vi "Calculate Frequency Response.vi"(9 "Amplitudes":dbl[](array[numeric]), 11 "Frequencies":dbl[](array[numeric])) -> (3 "Frequency response @ 1KHz":dbl[](array[numeric]))   [LabVIEW 2021, in "audio_frequencyResponseMeasurement.lvlib"]
uses:
  audio_frequencyResponseMeasurement.lvlib
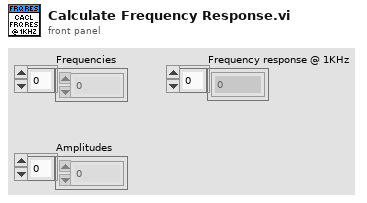
[diagram p1: front panel]
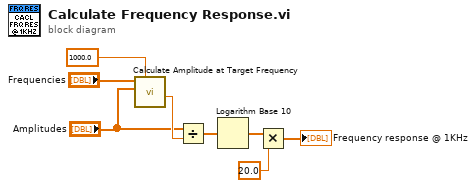
[diagram p0: block diagram]
diagram:
  n1 = call "Calculate Amplitude at Target Frequency.vi"("Target frequency"=1000.0, "Amplitudes"="Amplitudes", "Frequencies"="Frequencies") -> ("Amplitude @ target frequency"=w4:dbl)  [unwired: 8 in]
  n2 = Divide(x="Amplitudes", y=w4) -> (x/y=w7:dbl[])
  n3 = Logarithm Base 10(1:w7) -> (0:w6:dbl[])
  n4 = Multiply(x=w6, y=20.0) -> (x*y=→"Frequency response @ 1KHz":dbl[])
